vi "h.ACQ.GetActiveFullSpectrumDutChannelNumbers.vi"(8 "error in":errorcluster, 11 "Connection ID In":refnum<k5>) -> (0 "error out":errorcluster, 3 "Connection ID Out":refnum<k5>)   [LabVIEW 2016, in "h.Library.lvlib"]
doc: "Use this vi to setup the data rate divider for streaming. (e.g., set to 10 to stream every 10th data set; set to 1 to stream every data set)\n\n<b>Connection ID In</b> - is a network connection refnum that uniquely identifies the TCP connection\n<b>Timeout</b> - specifies the maximum amount of time, in milliseconds, for the function to complete\n<b>Data Rate Divider</b> - sets the interleave for data streaming \n<b>error in</b> - describes error conditions that occur before this node runs. This input provides standard\n<b>Connection ID Out</b> - returns the same value as connection ID\n<b>error out</b> - contains error information. This output provides standard error out functionality."
uses:
  h.Library.lvlib
panel:
  out "Active Channels":u32[](array[numeric])
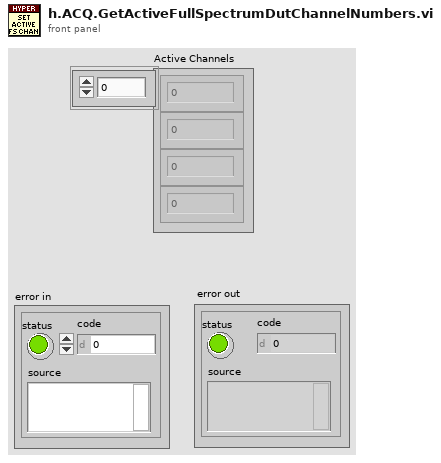
[diagram p1: front panel]
types:
  T1 = enum16{"big-endian, network order", "native, host order", "little-endian"}
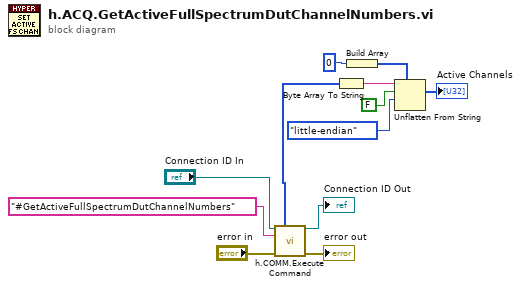
[diagram p0: block diagram]
diagram:
  n1 = call "h.COMM.Execute Command.vi"("Connection ID"="Connection ID In", "Command"="#GetActiveFullSpectrumDutChannelNumbers", "error in"="error in") -> ("Content"=w7:u8[], "Connection ID out"=→"Connection ID Out":refnum<k5>, "error out"=→"error out":errorcluster)  [unwired: 5 in, 5 out]
  n2 = Byte Array To String(unsigned byte array=w7) -> (string=w6:string)
  n3 = Build Array(u32 0) -> (w2:u32[])
  n4 = Unflatten From String(type=w2, binary string=w6, data includes array or string size? (T)=FALSE, byte order (0:big-endian, network order)=T1."little-endian") -> (value=→"Active Channels":u32[])  [unwired: 1 in, 2 out]
